vi "CreateHandleByGenTL.vi"(0 "error in (no error)":errorcluster caption="错误输入（无错误）", 1 "pDevInfo":T1) -> (2 "error out":errorcluster caption="错误输出", 3 "function return":i32 format="%x", 4 "handle":u64)   [LabVIEW 2015, in "MvCameraControl.lvlib"]
doc: "MV_LV_API int __stdcall CreateHandle(void ** handle, const MV_CC_DEVICE_INFO* pstDevInfo);"
uses:
  MvCameraControl.lvlib
  MvCameraPatch.dll
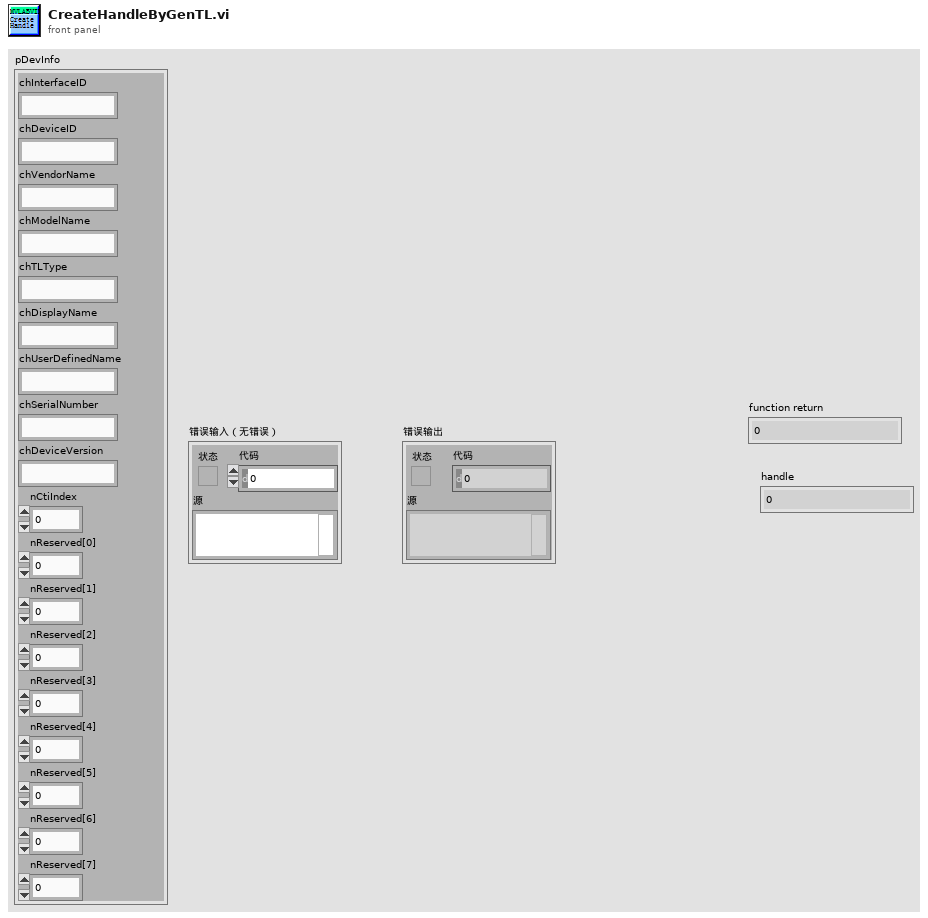
[diagram p1: front panel]
types:
  T1 = cluster{"chInterfaceID":string, "chDeviceID":string, "chVendorName":string, "chModelName":string, "chTLType":string, "chDisplayName":string, "chUserDefinedName":string, "chSerialNumber":string, "chDeviceVersion":string, "nCtiIndex":u32, "nReserved[0]":u32, "nReserved[1]":u32, "nReserved[2]":u32, "nReserved[3]":u32, "nReserved[4]":u32, "nReserved[5]":u32, "nReserved[6]":u32, "nReserved[7]":u32}
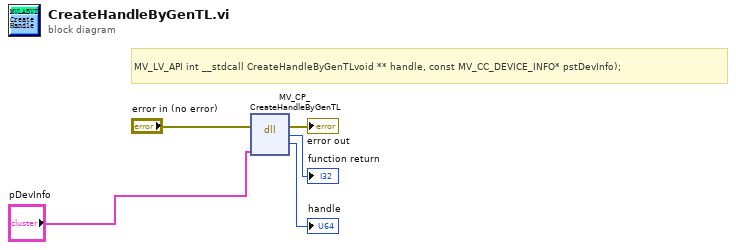
[diagram p0: block diagram]
diagram:
  # "MV_LV_API int __stdcall CreateHandleByGenTLvoid ** handle, const MV_CC_DEVICE_INFO* pstDevInfo);"
  n1 = dll-call lib="MvCameraPatch.dll" fn="MV_CP_CreateHandleByGenTL"(error in="error in (no error)", "pstDevInfo"="pDevInfo") -> (error out=→"error out":errorcluster, "返回类型"=→"function return":i32, "handle"=→"handle":u64)  [unwired: 4 in, 1 out]
